vi "FPGA_trigger_start.vi"(7 "Pulse params":T2, 8 "error in":errorcluster, 9 "TL Input":bool, 10 "Use Cont. trigger":bool, 11 "FPGA VI Reference IN":T1) -> (0 "error out":errorcluster)   [LabVIEW 2020]
uses:
  Standalone FPGA/FPGA_ref.ctl
  <vilib>/Utility/error.llb/Error Cluster From Error Code.vi
  <vilib>/rvi/errors/niLvFpgaAdjustHostInterfaceError.vi
  <vilib>/rvi/interface/nirviReadWriteControl/nirviReadWriteControl.xnode
  NiFpgaLv.dll
  <vilib>/rvi/interface/Simulation/niFpgaSimulationCallBeginRW.vi
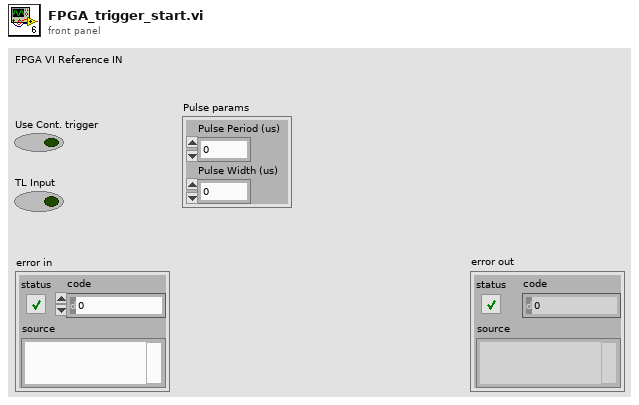
[diagram p1: front panel]
types:
  T1 = typedef "FPGA_ref.ctl" = refnum<k20>
  T2 = cluster{"Pulse Period (us)":u32, "Pulse Width (us)":u32}
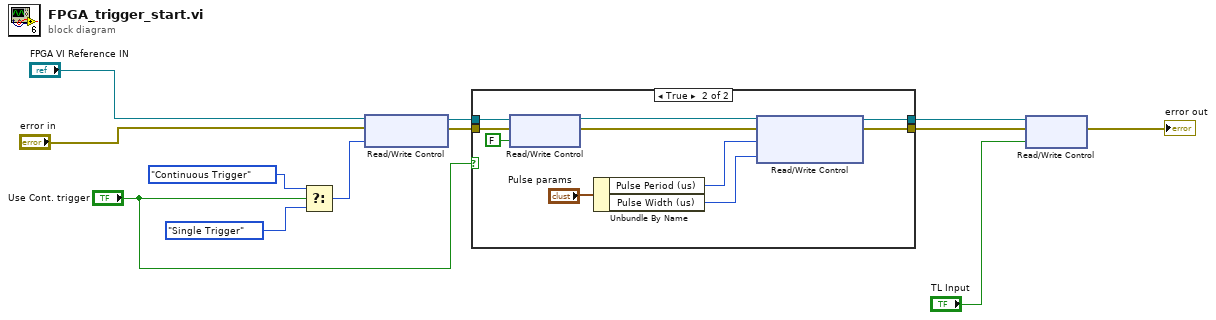
[diagram p0: block diagram]
diagram:
  n1 = Select(t=enum16{"Single Trigger", "Continuous Trigger"}."Continuous Trigger" ("Trigger Type"), s="Use Cont. trigger", f=enum16{"Single Trigger", "Continuous Trigger"}."Single Trigger" ("Trigger Type")) -> (s? t:f=w10:enum16{"Single Trigger", "Continuous Trigger"})
  n2 = xnode "Read/Write Control"("FPGA VI Reference In"="FPGA VI Reference IN", "error in"="error in", "Trigger Type"=w10) -> ("FPGA VI Reference Out"=w9:T1, "error out"=w8:errorcluster)
  n3 = case shown="True" "Use Cont. trigger" {
    tunnel: w9 -> [w14 w21]
    tunnel: w8 -> [w13 w20]
    tunnel: [w13 w16] -> w3
    tunnel: [w14 w15] -> w4
    frame False {
    }
    frame True {
      n4 = xnode "Read/Write Control"("FPGA VI Reference In"=w21, "error in"=w20, "stop_train"=FALSE) -> ("FPGA VI Reference Out"=w18:T1, "error out"=w17:errorcluster)
      n5 = Unbundle By Name("Pulse params") -> ("Pulse Period (us)"=w23:u32, "Pulse Width (us)"=w22:u32)
      n6 = xnode "Read/Write Control"("FPGA VI Reference In"=w18, "error in"=w17, "Pulse Period (us)"=w23, "Pulse Width (us)"=w22) -> ("FPGA VI Reference Out"=w15:T1, "error out"=w16:errorcluster)
    }
  }
  n7 = xnode "Read/Write Control"("FPGA VI Reference In"=w4, "error in"=w3, "TL Input"="TL Input") -> ("error out"=→"error out":errorcluster)  [unwired: 1 out]
